vi "ReadVersion.vi"(0 "VISA Refnum in":refnum<visa-resource-name>, 2 "Address":u8, 3 "error in (no error)":errorcluster) -> (5 "VISA Refnum out":refnum<visa-resource-name>, 6 "valid":bool, 7 "read buffer":string, 8 "error out":errorcluster)   [LabVIEW 2015, in "Ion Motion Roboclaw.lvlib"]
uses:
  <instrlib>/Ion Motion Roboclaw/Ion Motion Roboclaw.lvlib
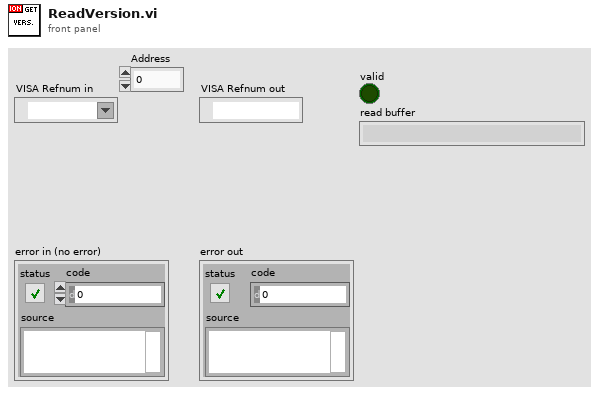
[diagram p1: front panel]
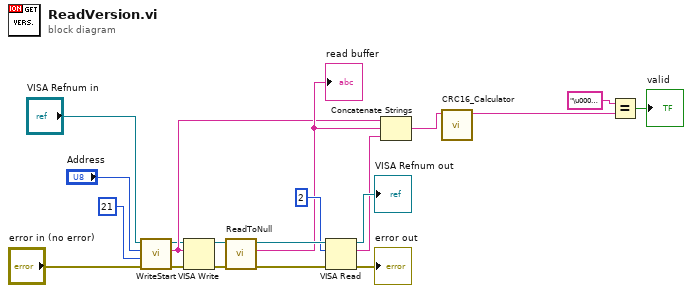
[diagram p0: block diagram]
diagram:
  n1 = call <instrlib>:"WriteStart.vi"("error in (no error)"="error in (no error)", "Cmd"=u8 21, "Address"="Address", "VISA Refnum in"="VISA Refnum in") -> ("error out"=w5:errorcluster, "String Out"=w7:string, "VISA Refnum out"=w6:refnum<visa-resource-name>)  [unwired: 5 in]
  n2 = VISA Write(VISA resource name=w6, write buffer=w7, error in (no error)=w5) -> (VISA resource name out=w4:refnum<visa-resource-name>, error out=w3:errorcluster)  [unwired: 1 out]
  n3 = call <instrlib>:"ReadToNull.vi"("error in (no error)"=w3, "VISA resource name"=w4) -> ("error out"=w20:errorcluster, "read buffer"=w15:string, "VISA resource name out"=w17:refnum<visa-resource-name>)  [unwired: 7 in]
  "read buffer" <- w15
  n4 = VISA Read(VISA resource name=w17, byte count=u32 2, error in (no error)=w20) -> (VISA resource name out=→"VISA Refnum out":refnum<visa-resource-name>, read buffer=w13:string, error out=→"error out":errorcluster)  [unwired: 1 out]
  n5 = Concatenate Strings(w7, w15, w13) -> (w14:string)
  n6 = call <instrlib>:"CRC16_Calculator.vi"("String in"=w14) -> ("CRC16 out"=w12:string)  [unwired: 8 in, 2 out]
  n7 = Equal?(x="\u0000\u0000", y=w12) -> (x = y?=→"valid":bool)
